vi "List Resources.vi"(8 "error in (no error)":errorcluster, 11 "RP2040.lvlib:RP2040Platform in":refnum<class "RP2040Platform.lvclass">) -> (0 "error out":errorcluster, 2 "Resources":refnum<class "Resource.lvclass">[](array[class]), 3 "RP2040.lvlib:RP2040Platform out":refnum<class "RP2040Platform.lvclass">)   [LabVIEW 2020, in "RP2040.lvlib" / "RP2040Platform.lvclass"]
uses:
  RP2040Platform.lvclass
  Builds/picoG/ppl/PicoG-Core.lvlibp/PicoG-Processor/PicoG-Core/Resource/Resource.lvclass
  Builds/picoG/ppl/PicoG-Core.lvlibp/PicoG-Processor/PicoG-Core/VisaResource/VisaResource.lvclass
  C:/dev/picoG/PicoG/Builds/picoG/ppl/PicoG-Core.lvlibp/PicoG-Processor/PicoG-Core/Resource/Resource.lvclass
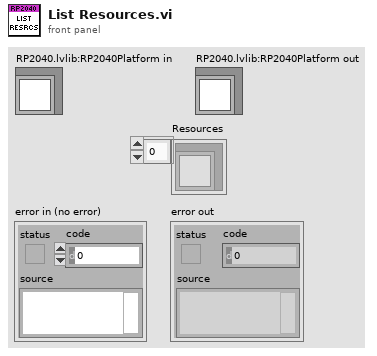
[diagram p1: front panel]
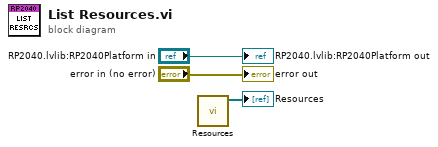
[diagram p0: block diagram]
diagram:
  n1 = call "Resources.vi"() -> ("Resources"=→"Resources":refnum<class "VisaResource.lvclass">[])  [unwired: 11 in]
  "error out" <- "error in (no error)"
  "RP2040.lvlib:RP2040Platform out" <- "RP2040.lvlib:RP2040Platform in"
